vi "Measurement UI.vi"() -> ()   [LabVIEW 2021, in "Waveform Mode_Channel Ganging UI.lvlib"]
uses:
  Waveform Mode_Channel Ganging UI.lvlib
  shared/UI/controls/view.ctl
panel:
  in  "MeasGraphs":enum32{"Results", "Hidden Controls"}(tab)
  in  "Current v/s Time":string="CURRENT v/s TIME"
  in  "Voltage v/s Time":string="VOLTAGE v/s TIME"
  in  "view current legend":T1
  in  "view voltage legend":T1
  out "CurrentGraph":waveform(dbl)[](graph) caption="AC"
  out "VoltageGraph":waveform(dbl)[](graph) caption="AC"
  in  "Mode of operation":T2(ring)
  out "Load dt":dbl[](array[numeric])
  in  "Load source delays":dbl[](array[numeric])
  in  "Load voltage/current setpoints":dbl[](array[numeric]) format="%#_6p"
  in  "Power ON/Source voltage/current setpoints":dbl[](array[numeric]) format="%#_6p"
  in  "Source source delays":dbl[](array[numeric])
  in  "Load voltage/current pole-zero ratios":dbl[](array[numeric])
  in  "Load voltage/current compensation frequencies":dbl[](array[numeric])
  in  "Load voltage/current gain bandwidths":dbl[](array[numeric])
  in  "Source voltage/current pole-zero ratios":dbl[](array[numeric])
  in  "Source voltage/current compensation frequencies":dbl[](array[numeric])
  in  "Source voltage/current gain bandwidths":dbl[](array[numeric])
  in  "Load resource names":string[](array[string])
  in  "Power ON/Source resource names":string[](array[string])
  out "Ganged load currents":dbl[](array[numeric])
  out "Ganged load voltages":dbl[](array[numeric])
  out "Ganged source currents":dbl[](array[numeric])
  out "Ganged source voltages":dbl[](array[numeric])
  out "Load currents":dbl[](array[numeric])
  out "Load voltages":dbl[](array[numeric])
  out "Source currents":dbl[](array[numeric])
  out "Source voltages":dbl[](array[numeric])
  out "Source dt":dbl[](array[numeric])
  in  "ModeOfConfiguration":T3(tab)
  in  "DEVICE POWER":bool=TRUE
  out "Status":string
  in  "Load config power on":string="Load Config"
  in  "POWERON/OFFLOADResourceNames":refnum<k15>[](array[refnum]) caption="RESOURCE NAMES\n(Single/Master & Slave)"
  in  "Source config power on":string="Source Config"
  in  "POWERON/OFFSOURCEResourceNames":refnum<k15>[](array[refnum]) caption="RESOURCE NAMES\n(Single/Master & Slave)"
  in  "Power on/off source sense":i32(ring)=1009 caption="SENSE" items=["Local"=1008, "Remote"=1009]
  in  "Power on/off Source voltage/current limit range":dbl=20.0 caption="CURRENT LIMIT" format="%#_6pA"
  in  "Power on/off Source voltage/current level":dbl=6.0 caption="VOLTAGE LEVEL" format="%#_6pV"
  in  "Power on/off source system configuration":enum32{"Series", "Parallel"}(ring)=enum."Parallel" caption="SYSTEM CONFIG"
  in  "Power on/off output function":i32(ring)=1006 caption="OUTPUT FUNCTION" items=["DC Voltage"=1006, "DC Current"=1007]
  out "Eload status":string
  in  "MeasConfigurations":enum32{"Source Config", "Load Config"}(tab)
  out "Source duration":string="            Duration"
  out "Source voltage/current":string="Voltage"
  in  "Source setpoints":T4(array[cluster]) {"Duration" format="%#_6ps"; "Voltage/Current Value" format="%#_6pV"}
  in  "Source timing":string="Timings"
  in  "Source aperture time":dbl=0.01666 caption="APERTURE TIME" format="%.3ps"
  in  "Source enable/disable":bool=TRUE caption="Source Enable/Disable"
  in  "PPSResourceNames":refnum<k15>[](array[refnum]) caption="RESOURCE NAMES\n(Single/Master & Slave)"
  in  "Source transient response":i32(ring)=1038 caption="TRANSIENT RESPONSE" items=["Slow"=1041, "Normal"=1038, "Fast"=1039, "Custom"=1042]
  in  "Power ON/Source sense":i32(ring)=1009 caption="SENSE" items=["Local"=1008, "Remote"=1009]
  in  "Source voltage/current level range":dbl=20.0 caption="VOLTAGE LEVEL RANGE" format="%#_6pV"
  in  "Source current/voltage limit high":dbl=25.0 caption="CURRENT LIMIT/LIMIT HIGH" format="%#_6pA"
  in  "Power ON/Source current/voltage limit range":dbl=25.0 caption="CURRENT LIMIT RANGE" format="%#_6pA"
  in  "Source limit symmetry":enum32{"Symmetric", "Asymmetric"}(ring)=enum."Asymmetric" caption="LIMIT SYMMETRY"
  in  "Source current/voltage limit low":dbl=-0.6 caption="CURRENT LIMIT LOW" format="%#_6pA"
  in  "Power ON/Source system configuration":enum32{"Series", "Parallel"}(ring)=enum."Parallel" caption="SYSTEM CONFIG"
  in  "Source compliance":string="Compliance"
  in  "Source sourceadapt":string="SourceAdapt"
  in  "Power ON/Source output function":i32(ring)=1006 caption="OUTPUT FUNCTION" items=["DC Voltage"=1006, "DC Current"=1007]
  in  "Source Custom Transient Response":bool
  in  "Load device voltage/current rating":dbl=30.0 caption="MAX CURRENT PER LOAD" format="%#_6pA"
  out "Load duration":string="            Duration"
  out "Load voltage/current":string="Current"
  in  "Load setpoints":T4(array[cluster]) {"Duration" format="%#_6ps"; "Voltage/Current Value" format="%#_6pA"}
  in  "Load aperture time":dbl=0.01666 caption="APERTURE TIME" format="%.3ps"
  in  "Load timing":string="Timings"
  in  "Load Custom Transient Response":bool
  in  "Load sourceadapt":string="SourceAdapt"
  in  "Load compliance":string="Compliance"
  in  "Load system configuration":enum32{"Series", "Parallel"}(ring)=enum."Parallel" caption="SYSTEM CONFIG"
  in  "Load current/voltage limit low":dbl caption="VOLTAGE  LIMIT LOW" format="%#_6pV"
  in  "Load limit symmetry":enum32{"Symmetric", "Asymmetric"}(ring) caption="LIMIT SYMMETRY"
  in  "Load current/voltage limit range":dbl=6.0 caption="VOLTAGE LIMIT RANGE" format="%#_6pV"
  in  "Load current/voltage limit high":dbl=inf caption="VOLTAGE LIMIT/LIMIT HIGH" format="%#_6p"
  in  "Load voltage/current level range":dbl=40.0 caption="CURRENT LEVEL RANGE" format="%#_6pA"
  in  "Load sense":i32(ring)=1009 caption="SENSE" items=["Local"=1008, "Remote"=1009]
  in  "Load transient response":i32(ring)=1038 caption="TRANSIENT RESPONSE" items=["Slow"=1041, "Normal"=1038, "Fast"=1039, "Custom"=1042]
  in  "Load output function":i32(ring)=1007 caption="OUTPUT FUNCTION" items=["DC Voltage"=1006, "DC Current"=1007]
  in  "Load enable/disable":bool caption="Load Enable/Disable"
  in  "LoadResourceNames":refnum<k15>[](array[refnum]) caption="RESOURCE NAMES\n(Single/Master & Slave)"
  # "V"
  # "I"
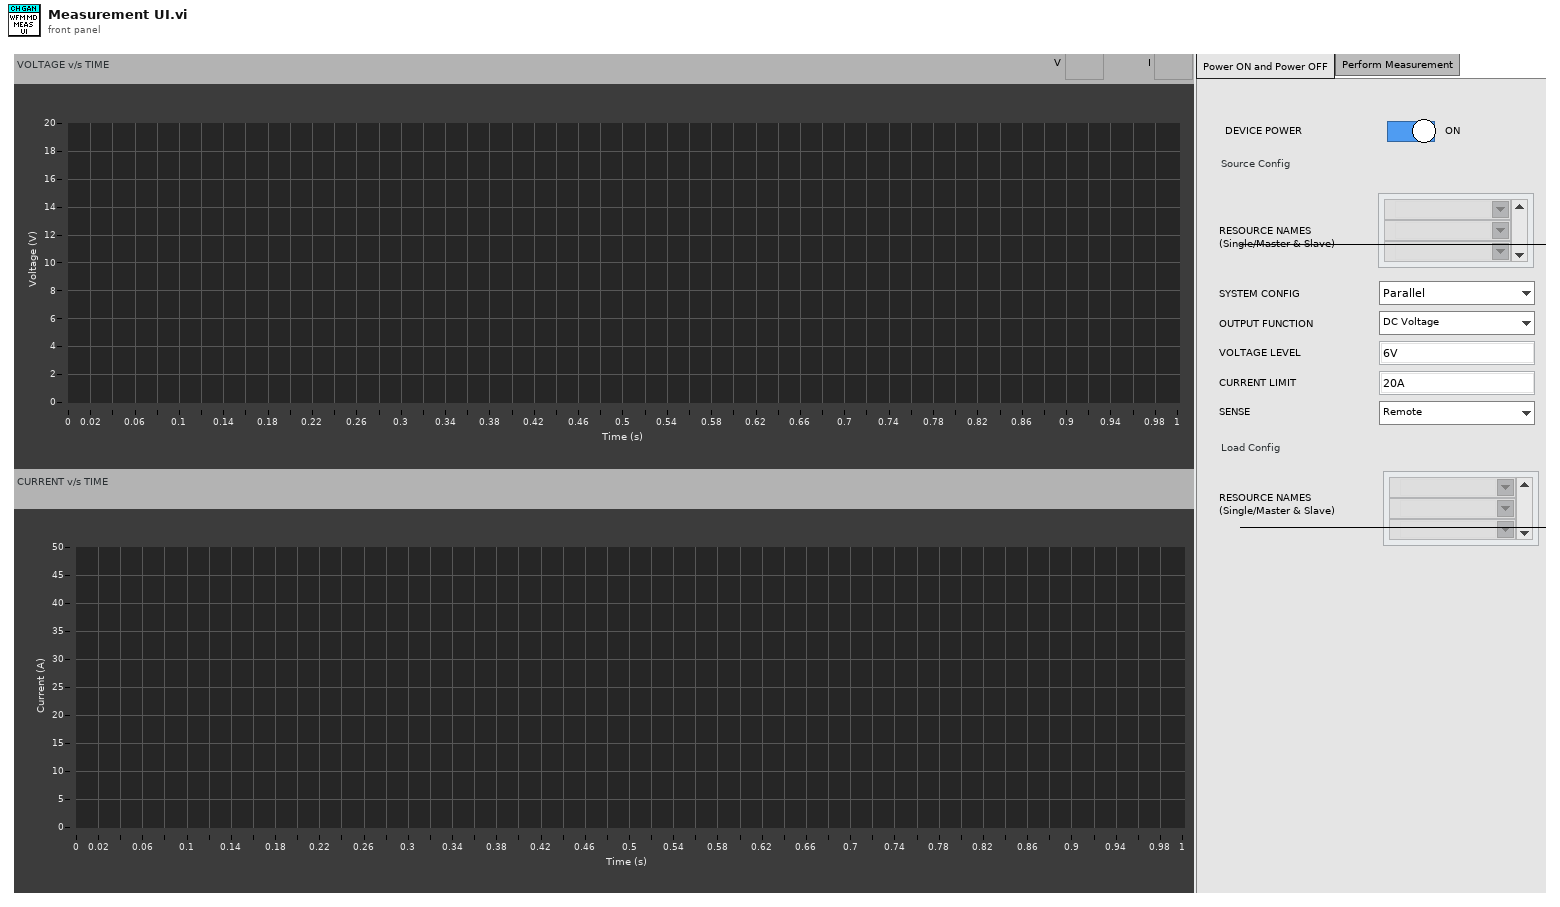
[diagram p1: front panel]
types:
  T1 = typedef "view.ctl" = bool
  T2 = enum32{"Power on the DUT", "Perform measurement", "Power off the DUT"}
  T3 = enum32{"Power ON and Power OFF", "Perform Measurement"}
  T4 = cluster{"Voltage/Current Value":dbl, "Duration":dbl}[]
  T5 = typedef "Multiple SourceAdapt Parameters.ctl" = cluster{"Voltage gain bandwidth":dbl, "Voltage compensation frequency":dbl, "Voltage pole-zero ratio":dbl, "Current gain bandwidth":dbl, "Current compensation frequency":dbl, "Current pole-zero ratio":dbl}[]
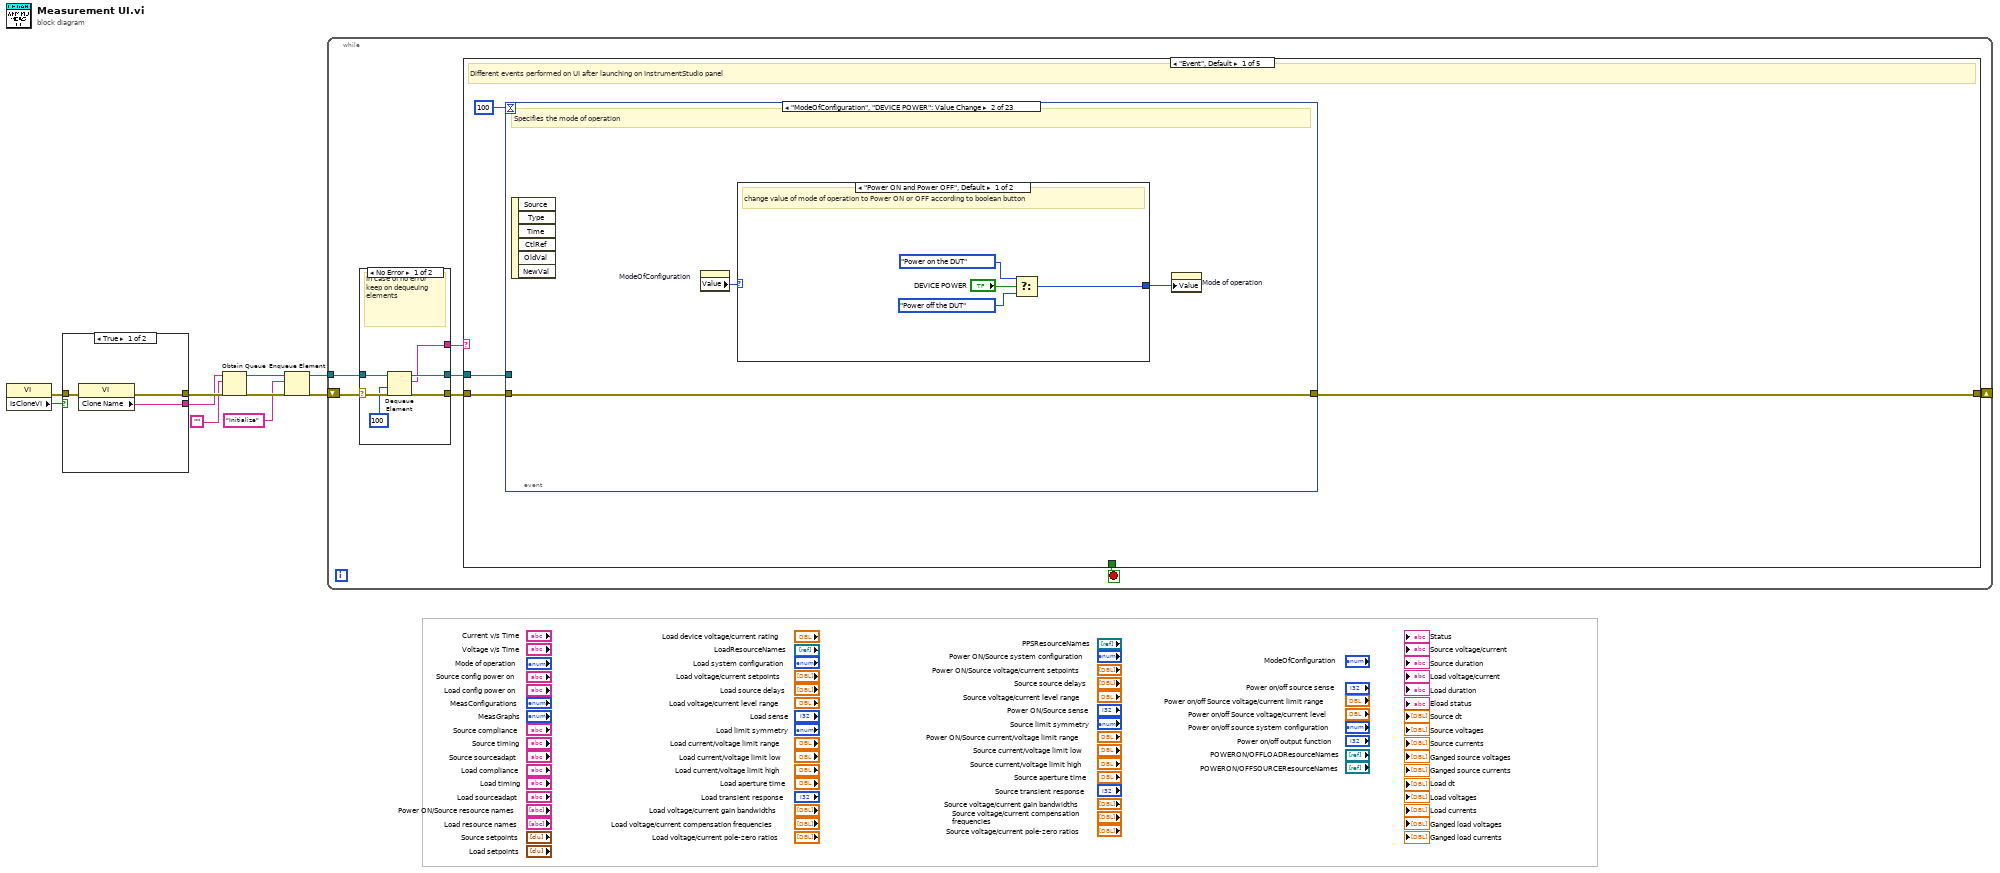
[diagram p0: block diagram]
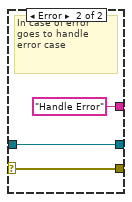
[diagram p2: hidden frame]
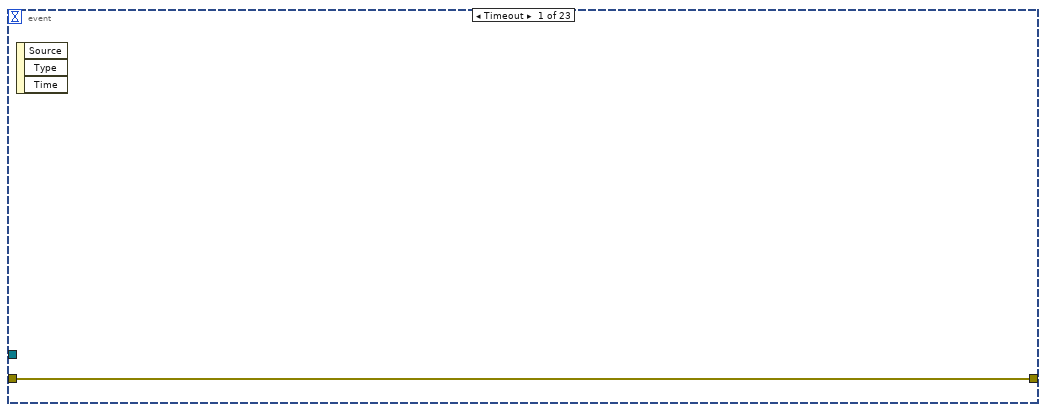
[diagram p3: hidden frame]
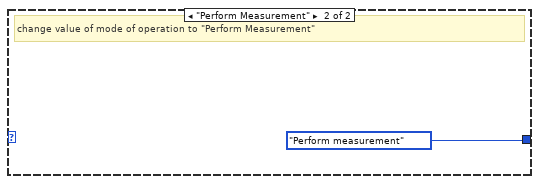
[diagram p4: hidden frame]
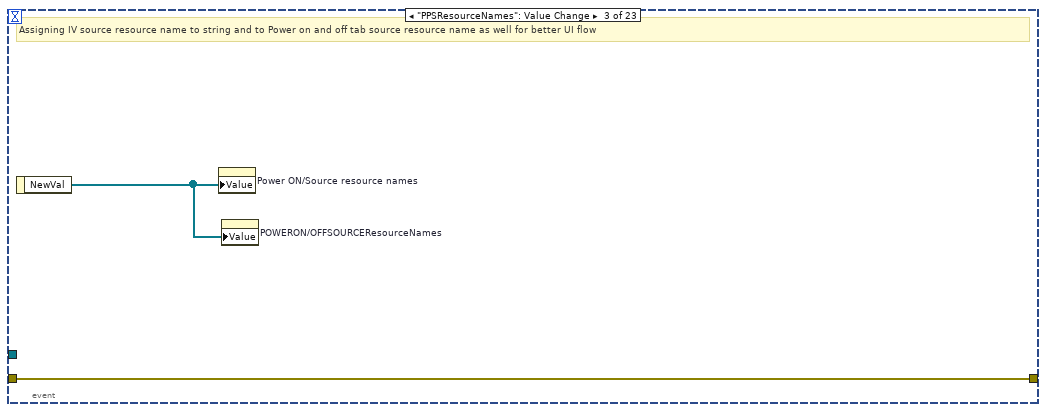
[diagram p5: hidden frame]
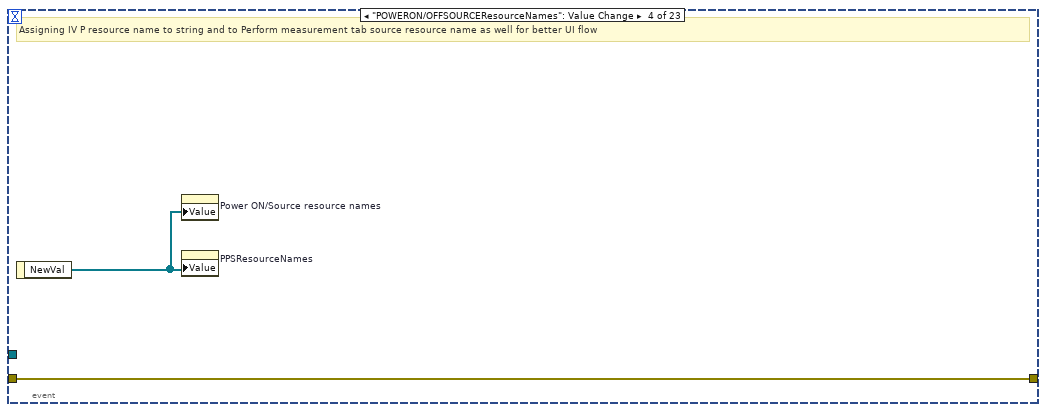
[diagram p6: hidden frame]
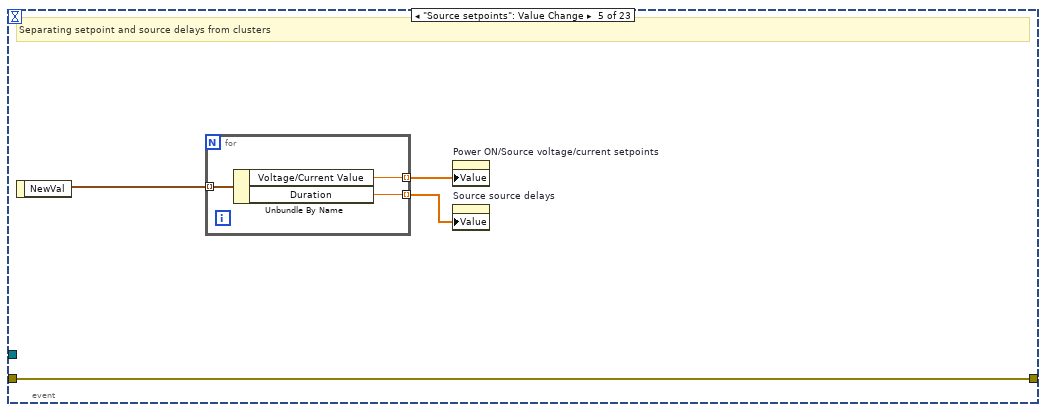
[diagram p7: hidden frame]
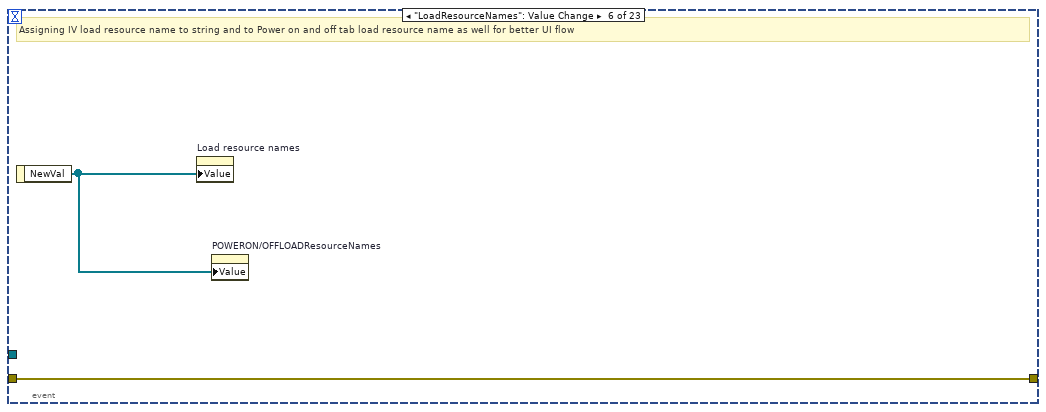
[diagram p8: hidden frame]
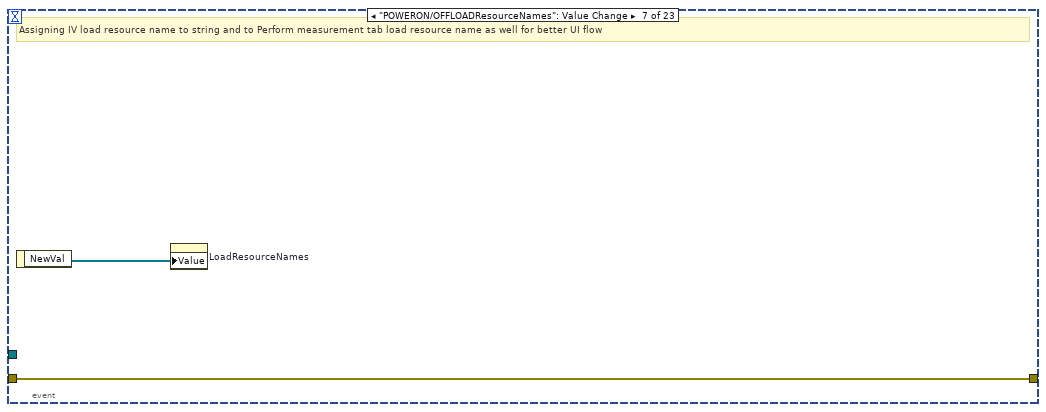
[diagram p9: hidden frame]
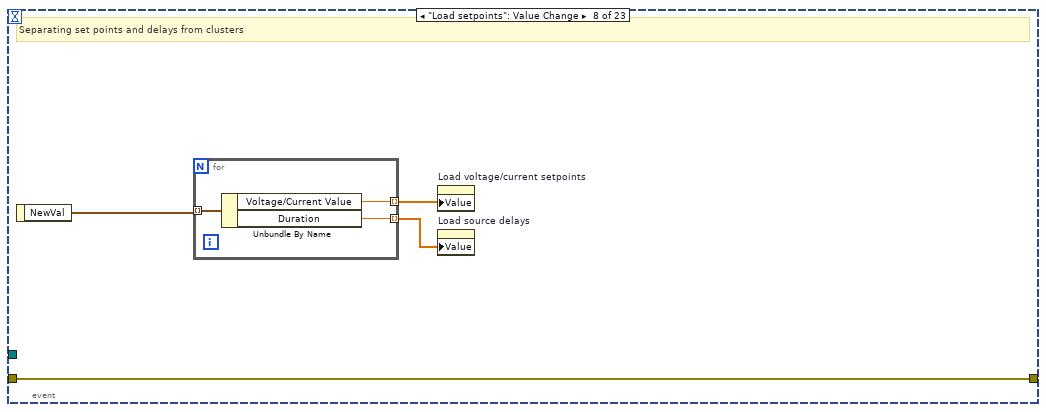
[diagram p10: hidden frame]
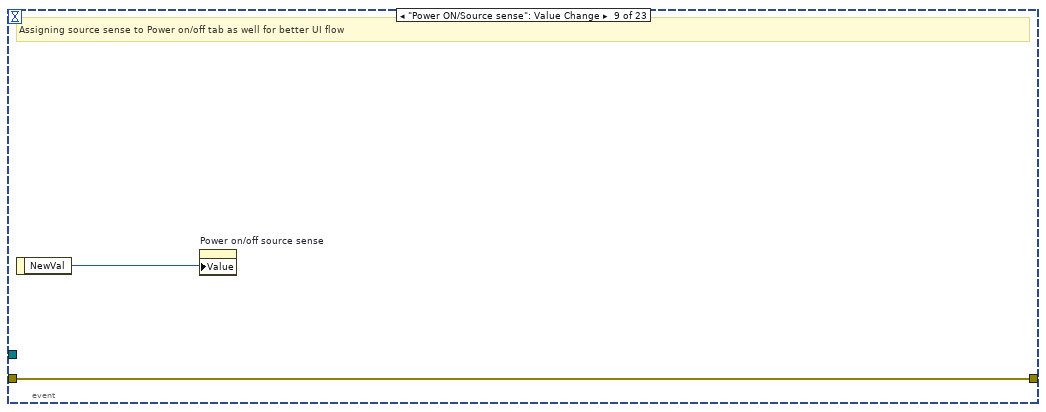
[diagram p11: hidden frame]
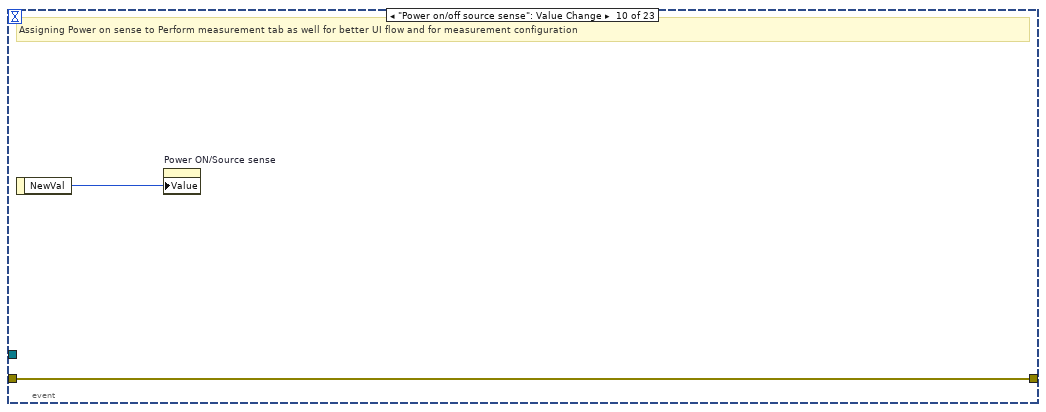
[diagram p12: hidden frame]
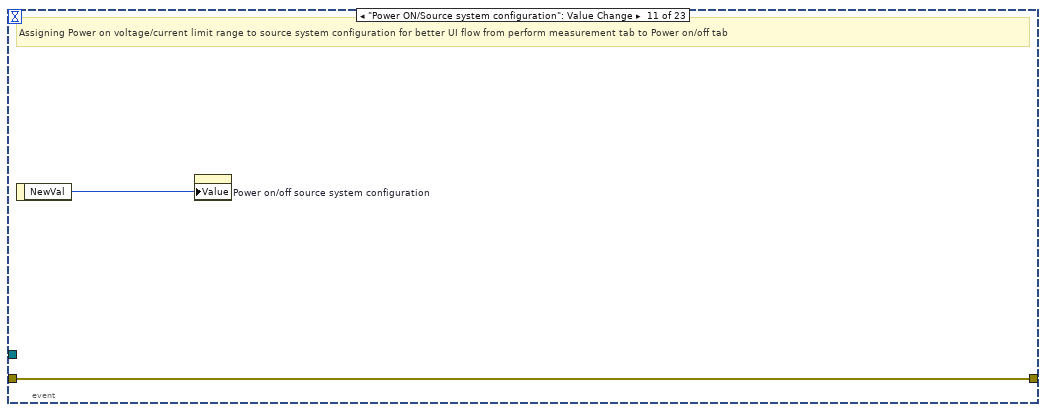
[diagram p13: hidden frame]
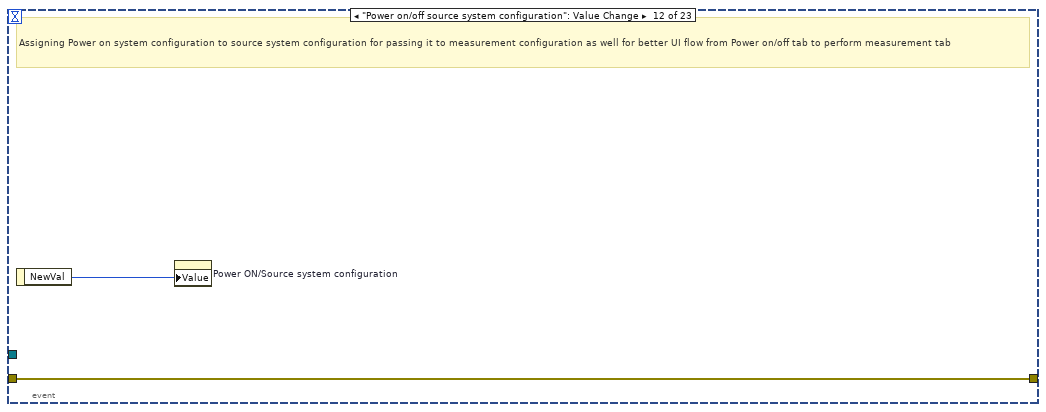
[diagram p14: hidden frame]
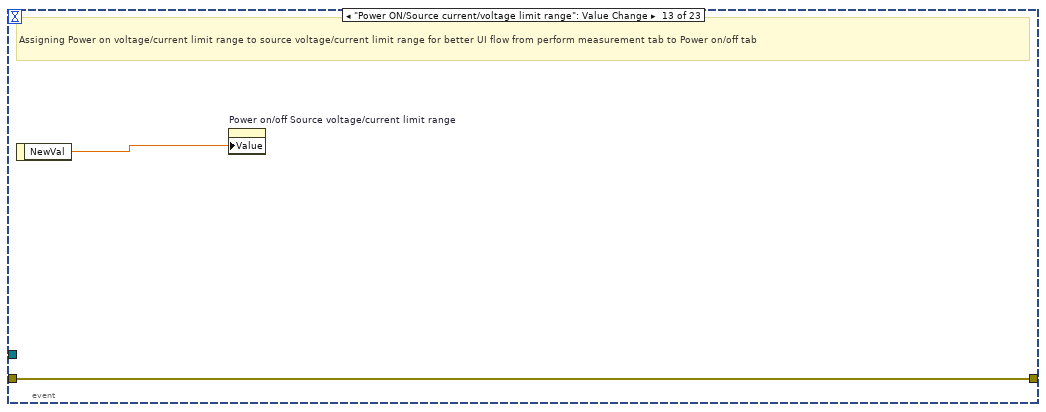
[diagram p15: hidden frame]
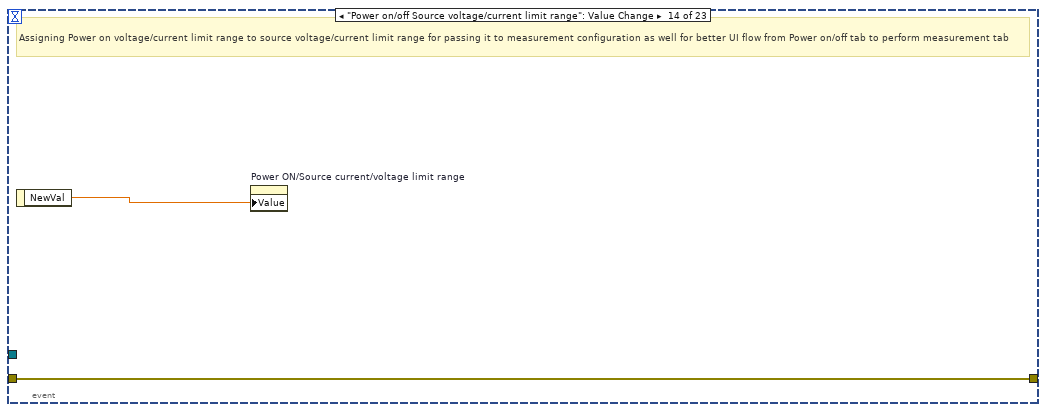
[diagram p16: hidden frame]
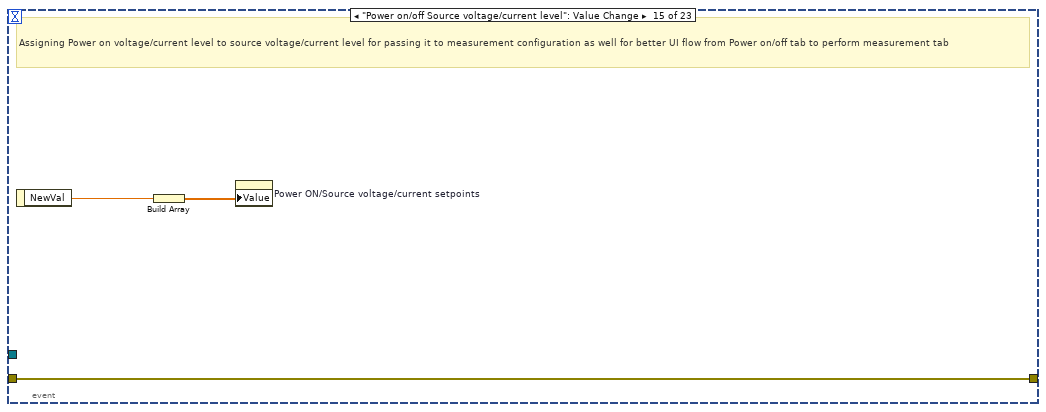
[diagram p17: hidden frame]
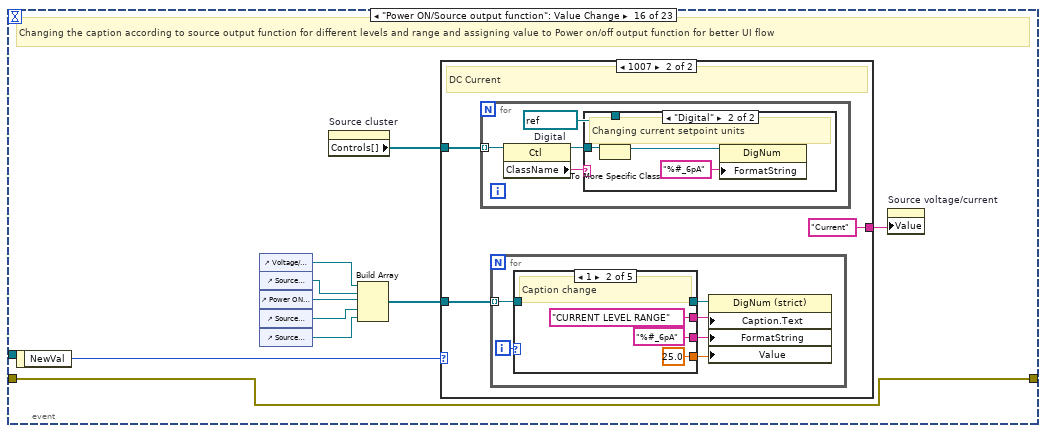
[diagram p18: hidden frame]
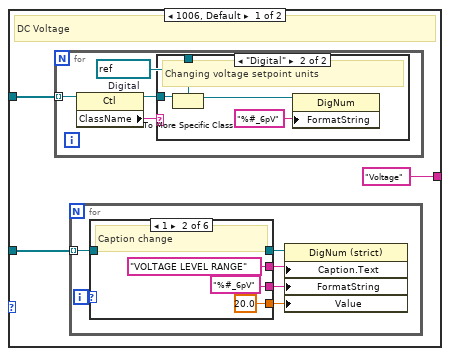
[diagram p19: hidden frame]
diagram:
  n1 = property class="VI"() -> (error out=w1:errorcluster, "IsCloneVI"=w2:bool)  [unwired: 2 in, 1 out]
  n2 = case shown="True" w2 {
    tunnel: [w13 w16] -> w10
    tunnel: [w12 w15] -> w9
    tunnel: w1 -> [w11 w14]
    frame True {
      n3 = property class="VI"(error in=w11) -> (error out=w13:errorcluster, "Clone Name"=w12:string)  [unwired: 1 in, 1 out]
    }
    frame False {
      n4 = property class="VI"(error in=w14) -> (error out=w16:errorcluster, "Name"=w15:string)  [unwired: 1 in, 1 out]
    }
  }
  n5 = Obtain Queue(name (unnamed)=w9, element data type="", error in (no error)=w10) -> (queue out=w6:refnum<queue>, error out=w8:errorcluster)  [unwired: 2 in, 1 out]
  n6 = Enqueue Element(queue=w6, element="Initialize", error in (no error)=w8) -> (queue out=w5:refnum<queue>, error out=w7:errorcluster)  [unwired: 1 in, 1 out]
  n7 = while {
    shift-right: [w18] -> _
    shift-left: w7 -> [w23]
    tunnel: w5 -> [w21]
    stop <- w17 stop-if-true
    n8 = case shown="No Error" w23 {
      selector: w23 -> [w29 w32]
      tunnel: [w28 w32] -> w22
      tunnel: w21 -> [w27 w31]
      tunnel: [w26 w31] -> w20
      tunnel: [w25 "Handle Error"] -> w19
      frame No Error {
        # "In case of no error keep on dequeuing elements"
        n9 = Dequeue Element(queue=w27, timeout in ms (-1)=100, error in (no error)=w29) -> (queue out=w26:refnum<queue>, element=w25:string, error out=w28:errorcluster)  [unwired: 1 out]
      }
      frame Error {
        # "In case of error goes to handle error case"
      }
    }
    n10 = case shown="\"Event\", Default" w19 {
      tunnel: w22 -> [w35 w348 w376 w470 w471]
      tunnel: w20 -> [w33 _ _ w468 _]
      tunnel: [w36 w348 w376 w465 w471] -> w18
      tunnel: [_ _ _ TRUE _] -> w17
      frame "Event", Default {
        # "Different events performed on UI after launching on InstrumentStudio panel"
        n11 = event shown="[1] \"ModeOfConfiguration\", \"DEVICE POWER\": Value Change" {
          selector: _ -> [_ _ _ _ _ _ _ _ _ _ _ _ _ _ _ _ _ _ _ _ _ _ _]
          dyn-events: _ -> [_ _ _ _ _ _ _ _ _ _ _ _ _ _ _ _ _ _ _ _ _ _ _]
          timeout: 100 -> [_ _ _ _ _ _ _ _ _ _ _ _ _ _ _ _ _ _ _ _ _ _ _]
          tunnel: [w37 w38 w47 w48 w52 w58 w59 w63 w68 w70 w72 w74 w76 w78 w80 w83 w165 w200 w286 w305 w319 w332 w345] -> w36
          tunnel: w35 -> [w37 w38 w47 w48 w52 w58 w59 w63 w68 w70 w72 w74 w76 w78 w80 w83 w165 w200 w286 w305 w320 w333 w346]
          tunnel: w33 -> [_ _ _ _ _ _ _ _ _ _ _ _ _ _ _ _ _ _ _ _ _ _ w344]
          event Timeout {
            n12 = event-data() -> ()  [unwired: 1 in, 3 out]
          }
          event "ModeOfConfiguration", "DEVICE POWER": Value Change {
            # "Specifies the mode of operation"
            n13 = event-data() -> ()  [unwired: 1 in, 6 out]
            n14 = property on="ModeOfConfiguration" class="TabCtl (strict)"() -> ("Value"=w40:T3)  [unwired: 2 in, 2 out]
            n15 = case shown="\"Power ON and Power OFF\", Default" w40 {
              tunnel: [w42 T2."Perform measurement" ("Mode of operation")] -> w39
              frame "Power ON and Power OFF", Default {
                # "change value of mode of operation to Power ON or OFF according to boolean button"
                n16 = Select(t=T2."Power on the DUT" ("Mode of operation"), s="DEVICE POWER", f=T2."Power off the DUT" ("Mode of operation")) -> (s? t:f=w42:T2)
              }
              frame "Perform Measurement" {
                # "change value of mode of operation to \"Perform Measurement\""
              }
            }
            n17 = property on="Mode of operation" class="Enum (strict)"("Value"=w39) -> ()  [unwired: 2 in, 2 out]
          }
          event "PPSResourceNames": Value Change {
            # "Assigning IV source resource name to string and to Power on and off tab source resource name as well for better UI flow"
            n18 = event-data() -> ("NewVal"=w46:refnum<k15>[])  [unwired: 1 in]
            n19 = property on="Power ON/Source resource names" class="Arr (strict)"("Value"=w46) -> ()  [unwired: 2 in, 2 out]
            n20 = property on="POWERON/OFFSOURCEResourceNames" class="Arr (strict)"("Value"=w46) -> ()  [unwired: 2 in, 2 out]
          }
          event "POWERON/OFFSOURCEResourceNames": Value Change {
            # "Assigning IV P resource name to string and to Perform measurement tab source resource name as well for better UI flow"
            n21 = event-data() -> ("NewVal"=w49:refnum<k15>[])  [unwired: 1 in]
            n22 = property on="Power ON/Source resource names" class="Arr (strict)"("Value"=w49) -> ()  [unwired: 2 in, 2 out]
            n23 = property on="PPSResourceNames" class="Arr (strict)"("Value"=w49) -> ()  [unwired: 2 in, 2 out]
          }
          event "Source setpoints": Value Change {
            # "Separating setpoint and source delays from clusters"
            n24 = event-data() -> ("NewVal"=w53:T4)  [unwired: 1 in]
            n25 = for {
              tunnel: w53 -> [w56] mode=indexing
              tunnel: [w55] -> w51 mode=indexing
              tunnel: [w54] -> w50 mode=indexing
              n26 = Unbundle By Name(w56) -> ("Voltage/Current Value"=w55:dbl, "Duration"=w54:dbl)
            }
            n27 = property on="Power ON/Source voltage/current setpoints" class="Arr (strict)"("Value"=w51) -> ()  [unwired: 2 in, 2 out]
            n28 = property on="Source source delays" class="Arr (strict)"("Value"=w50) -> ()  [unwired: 2 in, 2 out]
          }
          event "LoadResourceNames": Value Change {
            # "Assigning IV load resource name to string and to Power on and off tab load resource name as well for better UI flow"
            n29 = event-data() -> ("NewVal"=w57:refnum<k15>[])  [unwired: 1 in]
            n30 = property on="Load resource names" class="Arr (strict)"("Value"=w57) -> ()  [unwired: 2 in, 2 out]
            n31 = property on="POWERON/OFFLOADResourceNames" class="Arr (strict)"("Value"=w57) -> ()  [unwired: 2 in, 2 out]
          }
          event "POWERON/OFFLOADResourceNames": Value Change {
            # "Assigning IV load resource name to string and to Perform measurement tab load resource name as well for better UI flow"
            n32 = event-data() -> ("NewVal"=w60:refnum<k15>[])  [unwired: 1 in]
            n33 = property on="LoadResourceNames" class="Arr (strict)"("Value"=w60) -> ()  [unwired: 2 in, 2 out]
          }
          event "Load setpoints": Value Change {
            # "Separating set points and delays from clusters"
            n34 = event-data() -> ("NewVal"=w64:T4)  [unwired: 1 in]
            n35 = for {
              tunnel: w64 -> [w67] mode=indexing
              tunnel: [w66] -> w62 mode=indexing
              tunnel: [w65] -> w61 mode=indexing
              n36 = Unbundle By Name(w67) -> ("Voltage/Current Value"=w66:dbl, "Duration"=w65:dbl)
            }
            n37 = property on="Load voltage/current setpoints" class="Arr (strict)"("Value"=w62) -> ()  [unwired: 2 in, 2 out]
            n38 = property on="Load source delays" class="Arr (strict)"("Value"=w61) -> ()  [unwired: 2 in, 2 out]
          }
          event "Power ON/Source sense": Value Change {
            # "Assigning source sense to Power on/off tab as well for better UI flow"
            n39 = event-data() -> ("NewVal"=w69:i32)  [unwired: 1 in]
            n40 = property on="Power on/off source sense" class="Ring (strict)"("Value"=w69) -> ()  [unwired: 2 in, 2 out]
          }
          event "Power on/off source sense": Value Change {
            # "Assigning Power on sense to Perform measurement tab as well for better UI flow and for measurement configuration"
            n41 = event-data() -> ("NewVal"=w71:i32)  [unwired: 1 in]
            n42 = property on="Power ON/Source sense" class="Ring (strict)"("Value"=w71) -> ()  [unwired: 2 in, 2 out]
          }
          event "Power ON/Source system configuration": Value Change {
            # "Assigning Power on voltage/current limit range to source system configuration for better UI flow from perform measurement tab to Power on/off tab"
            n43 = event-data() -> ("NewVal"=w73:enum32{"Series", "Parallel"})  [unwired: 1 in]
            n44 = property on="Power on/off source system configuration" class="Enum (strict)"("Value"=w73) -> ()  [unwired: 2 in, 2 out]
          }
          event "Power on/off source system configuration": Value Change {
            # "Assigning Power on system configuration to source system configuration for passing it to measurement configuration as well for better UI flow from Power on/off tab to perform measurement tab"
            n45 = event-data() -> ("NewVal"=w75:enum32{"Series", "Parallel"})  [unwired: 1 in]
            n46 = property on="Power ON/Source system configuration" class="Enum (strict)"("Value"=w75) -> ()  [unwired: 2 in, 2 out]
          }
          event "Power ON/Source current/voltage limit range": Value Change {
            # "Assigning Power on voltage/current limit range to source voltage/current limit range for better UI flow from perform measurement tab to Power on/off tab"
            n47 = event-data() -> ("NewVal"=w77:dbl)  [unwired: 1 in]
            n48 = property on="Power on/off Source voltage/current limit range" class="DigNum (strict)"("Value"=w77) -> ()  [unwired: 2 in, 2 out]
          }
          event "Power on/off Source voltage/current limit range": Value Change {
            # "Assigning Power on voltage/current limit range to source voltage/current limit range for passing it to measurement configuration as well for better UI flow from Power on/off tab to perform measurement tab"
            n49 = event-data() -> ("NewVal"=w79:dbl)  [unwired: 1 in]
            n50 = property on="Power ON/Source current/voltage limit range" class="DigNum (strict)"("Value"=w79) -> ()  [unwired: 2 in, 2 out]
          }
          event "Power on/off Source voltage/current level": Value Change {
            # "Assigning Power on voltage/current level to source voltage/current level for passing it to measurement configuration as well for better UI flow from Power on/off tab to perform measurement tab"
            n51 = event-data() -> ("NewVal"=w82:dbl)  [unwired: 1 in]
            n52 = Build Array(w82) -> (w81:dbl[])
            n53 = property on="Power ON/Source voltage/current setpoints" class="Arr (strict)"("Value"=w81) -> ()  [unwired: 2 in, 2 out]
          }
          event "Power ON/Source output function": Value Change {
            # "Changing the caption according to source output function for different levels and range and assigning value to Power on/off output function for better UI flow"
            n54 = event-data() -> ("NewVal"=w92:i32)  [unwired: 1 in]
            n55 = control-ref of="Voltage/Current Value"() -> (w86:refnum<vi>)
            n56 = control-ref of="Source voltage/current level range"() -> (w91:refnum<vi>)
            n57 = control-ref of="Power ON/Source current/voltage limit range"() -> (w90:refnum<vi>)
            n58 = control-ref of="Source current/voltage limit low"() -> (w89:refnum<vi>)
            n59 = control-ref of="Source current/voltage limit high"() -> (w88:refnum<vi>)
            n60 = property on="Source cluster" class="Clust (strict)"() -> ("Controls[]"=w85:refnum<vi>[])  [unwired: 2 in, 2 out]
            n61 = Build Array(w86, w91, w90, w89, w88) -> (w87:refnum<vi>[])
            n62 = case shown="1007" w92 {
              tunnel: w87 -> [w95 w129]
              tunnel: w85 -> [w94 w128]
              tunnel: ["Voltage" ("Source voltage/current") "Current" ("Source voltage/current")] -> w84
              frame 1006, Default {
                # "DC Voltage"
                n63 = for {
                  tunnel: w94 -> [w99] mode=indexing
                  w97 = refnum<vi> refnum  # Digital
                  n64 = property class="Ctl"(reference=w99) -> (reference out=w98:refnum<vi>, "ClassName"=w96:string)  [unwired: 1 in, 1 out]
                  n65 = case shown="\"Digital\"" w96 {
                    tunnel: w98 -> [_ w103]
                    tunnel: w97 -> [_ w102]
                    frame Default {
                    }
                    frame "Digital" {
                      # "Changing voltage setpoint units"
                      n66 = To More Specific Class(target class=w102, reference=w103) -> (specific class reference=w101:refnum<vi>)  [unwired: 1 in, 1 out]
                      n67 = property class="DigNum"(reference=w101, "FormatString"="%#_6pV" ("Format String")) -> ()  [unwired: 1 in, 2 out]
                    }
                  }
                }
                n68 = for {
                  tunnel: w95 -> [w107] mode=indexing
                  i -> [w109]
                  n69 = case shown="1" w109 {
                    tunnel: [w110 w114 w118 w121 w125 _] -> w108
                    tunnel: w107 -> [w110 w114 w118 w121 w125 _]
                    tunnel: [_ "VOLTAGE LEVEL RANGE" ("Caption.Text") "CURRENT LIMIT RANGE" ("Caption.Text") "CURRENT LIMIT LOW" ("Caption.Text") "CURRENT LIMIT/LIMIT HIGH" ("Caption.Text") _] -> w106
                    tunnel: [_ "%#_6pV" ("Format String") "%#_6pA" ("Format String") "%#_6pA" ("Format String") "%#_6pA" ("Format String") _] -> w105
                    tunnel: [_ 20.0 ("Value") 25.0 ("Value") -0.6 ("Value") 25.0 ("Value") _] -> w104
                    frame 0 {
                    }
                    frame 1 {
                      # "Caption change"
                    }
                    frame 2 {
                      # "Caption change"
                    }
                    frame 3 {
                      # "Caption change"
                    }
                    frame 4 {
                      # "Caption change"
                    }
                    frame Default {
                    }
                  }
                  n70 = property class="DigNum (strict)"(reference=w108, "Caption.Text"=w106, "FormatString"=w105, "Value"=w104) -> ()  [unwired: 1 in, 2 out]
                }
              }
              frame 1007 {
                # "DC Current"
                n71 = for {
                  tunnel: w128 -> [w133] mode=indexing
                  w131 = refnum<vi> refnum  # Digital
                  n72 = property class="Ctl"(reference=w133) -> (reference out=w132:refnum<vi>, "ClassName"=w130:string)  [unwired: 1 in, 1 out]
                  n73 = case shown="\"Digital\"" w130 {
                    tunnel: w132 -> [_ w137]
                    tunnel: w131 -> [_ w136]
                    frame Default {
                    }
                    frame "Digital" {
                      # "Changing current setpoint units"
                      n74 = To More Specific Class(target class=w136, reference=w137) -> (specific class reference=w135:refnum<vi>)  [unwired: 1 in, 1 out]
                      n75 = property class="DigNum"(reference=w135, "FormatString"="%#_6pA" ("Format String")) -> ()  [unwired: 1 in, 2 out]
                    }
                  }
                }
                n76 = for {
                  tunnel: w129 -> [w141] mode=indexing
                  i -> [w143]
                  n77 = case shown="1" w143 {
                    tunnel: [w144 w148 w152 w155 w159] -> w142
                    tunnel: w141 -> [w144 w148 w152 w155 w159]
                    tunnel: [_ "CURRENT LEVEL RANGE" ("Caption.Text") "VOLTAGE LIMIT RANGE" ("Caption.Text") "VOLTAGE  LIMIT LOW" ("Caption.Text") "VOLTAGE LIMIT/LIMIT HIGH" ("Caption.Text")] -> w140
                    tunnel: [_ "%#_6pA" ("Format String") "%#_6pV" ("Format String") "%#_6pV" ("Format String") "%#_6pV" ("Format String")] -> w139
                    tunnel: [_ 25.0 ("Value") 20.0 ("Value") -0.6 ("Value") 20.0 ("Value")] -> w138
                    frame 0, Default {
                    }
                    frame 1 {
                      # "Caption change"
                    }
                    frame 2 {
                      # "Caption change"
                    }
                    frame 3 {
                      # "Caption change"
                    }
                    frame 4 {
                      # "Caption change"
                    }
                  }
                  n78 = property class="DigNum (strict)"(reference=w142, "Caption.Text"=w140, "FormatString"=w139, "Value"=w138) -> ()  [unwired: 1 in, 2 out]
                }
              }
            }
            n79 = property on="Source voltage/current" class="Str"("Value"=w84) -> ()  [unwired: 2 in, 2 out]
          }
          event "Power on/off output function": Value Change {
            # "Assigning Power on output function to source output function for passing it to measurement configuration as well for better UI flow"
            n80 = event-data() -> ("NewVal"=w164:i32)  [unwired: 1 in]
            n81 = property on="Power ON/Source output function" class="Ring (strict)"("Value"=w164) -> ()  [unwired: 2 in, 2 out]
            n82 = control-ref of="Power on/off Source voltage/current level"() -> (w161:refnum<vi>)
            n83 = control-ref of="Power on/off Source voltage/current limit range"() -> (w162:refnum<vi>)
            n84 = Build Array(w162, w161) -> (w163:refnum<vi>[])
            n85 = case shown="1006, Default" w164 {
              tunnel: w163 -> [w167 w184]
              tunnel: [w166 w183] -> _
              frame 1006, Default {
                # "DC Voltage"
                n86 = for {
                  tunnel: w167 -> [w172] mode=indexing
                  tunnel: [w168] -> w166 mode=indexing
                  i -> [w174]
                  n87 = case shown="0, 2" w174 {
                    tunnel: [w178 w182 _] -> w173
                    tunnel: w172 -> [w178 w182 _]
                    tunnel: ["VOLTAGE LEVEL" ("Caption.Text") "CURRENT LIMIT" ("Caption.Text") _] -> w171
                    tunnel: ["%#_6pV" ("Format String") "%#_6pA" ("Format String") _] -> w170
                    tunnel: [6.0 ("Value") 20.0 ("Value") _] -> w169
                    frame 1 {
                      # "Voltage level cap change"
                    }
                    frame 0, 2 {
                      # "Current limit cap change"
                    }
                    frame Default {
                    }
                  }
                  n88 = property class="DigNum (strict)"(reference=w173, "Caption.Text"=w171, "FormatString"=w170, "Value"=w169) -> (reference out=w168:refnum<vi>)  [unwired: 1 in, 1 out]
                }
              }
              frame 1007 {
                # "DC Current"
                n89 = for {
                  tunnel: w184 -> [w189] mode=indexing
                  tunnel: [w185] -> w183 mode=indexing
                  i -> [w191]
                  n90 = case shown="1" w191 {
                    tunnel: [w195 w199 _] -> w190
                    tunnel: w189 -> [w195 w199 _]
                    tunnel: ["CURRENT LEVEL" ("Caption.Text") "VOLTAGE LIMIT" ("Caption.Text") _] -> w188
                    tunnel: ["%#_6pA" ("Format String") "%#_6pV" ("Format String") _] -> w187
                    tunnel: [10.0 ("Value") 20.0 ("Value") _] -> w186
                    frame 1 {
                      # "Current level cap change"
                    }
                    frame 0, 2 {
                      # "Voltage limit cap change"
                    }
                    frame Default {
                    }
                  }
                  n91 = property class="DigNum (strict)"(reference=w190, "Caption.Text"=w188, "FormatString"=w187, "Value"=w186) -> (reference out=w185:refnum<vi>)  [unwired: 1 in, 1 out]
                }
              }
            }
          }
          event "Load output function": Value Change {
            # "Changing reference according to Load output function DC Current or DC voltage"
            n92 = event-data() -> ("NewVal"=w201:i32)  [unwired: 1 in]
            n93 = property on="Power on/off output function" class="Ring (strict)"("Value"=w201) -> ()  [unwired: 2 in, 2 out]
            n94 = control-ref of="Voltage/Current Value"() -> (w204:refnum<vi>)
            n95 = control-ref of="Load voltage/current level range"() -> (w209:refnum<vi>)
            n96 = control-ref of="Load current/voltage limit range"() -> (w208:refnum<vi>)
            n97 = control-ref of="Load current/voltage limit low"() -> (w207:refnum<vi>)
            n98 = control-ref of="Load current/voltage limit high"() -> (w206:refnum<vi>)
            n99 = property on="Load cluster" class="Clust (strict)"() -> ("Controls[]"=w203:refnum<vi>[])  [unwired: 2 in, 2 out]
            n100 = Build Array(w204, w209, w208, w207, w206) -> (w205:refnum<vi>[])
            n101 = case shown="1007, Default" w201 {
              tunnel: w205 -> [w213 w248]
              tunnel: w203 -> [w211 w246]
              tunnel: ["Voltage" ("Load voltage/current") "Current" ("Load voltage/current")] -> w202
              frame 1006 {
                # "DC Voltage"
                n102 = for {
                  N: 1 -> [_]
                  tunnel: w211 -> [w217] mode=indexing
                  w215 = refnum<vi> refnum  # Digital
                  n103 = property class="Ctl"(reference=w217) -> (reference out=w216:refnum<vi>, "ClassName"=w214:string)  [unwired: 1 in, 1 out]
                  n104 = case shown="\"Digital\"" w214 {
                    tunnel: w216 -> [_ w221]
                    tunnel: w215 -> [_ w220]
                    frame Default {
                    }
                    frame "Digital" {
                      # "Changing voltage setpoint units"
                      n105 = To More Specific Class(target class=w220, reference=w221) -> (specific class reference=w219:refnum<vi>)  [unwired: 1 in, 1 out]
                      n106 = property class="DigNum"(reference=w219, "FormatString"="%#_6pV" ("Format String")) -> ()  [unwired: 1 in, 2 out]
                    }
                  }
                }
                n107 = for {
                  tunnel: w213 -> [w225] mode=indexing
                  i -> [w227]
                  n108 = case shown="1" w227 {
                    tunnel: [w228 w232 w236 w239 w243 _] -> w226
                    tunnel: w225 -> [w228 w232 w236 w239 w243 _]
                    tunnel: [_ "VOLTAGE LEVEL RANGE" ("Caption.Text") "CURRENT LIMIT RANGE" ("Caption.Text") "CURRENT LIMIT LOW" ("Caption.Text") "CURRENT LIMIT/LIMIT HIGH" ("Caption.Text") _] -> w224
                    tunnel: [_ "%#_6pV" ("Format String") "%#_6pA" ("Format String") "%#_6pA" ("Format String") "%#_6pA" ("Format String") _] -> w223
                    tunnel: [_ 6.0 ("Value") 40.0 ("Value") 0.0 ("Value") 40.0 ("Value") _] -> w222
                    frame 0 {
                    }
                    frame 1 {
                      # "Caption change"
                    }
                    frame 2 {
                      # "Caption change"
                    }
                    frame 3 {
                      # "Caption change"
                    }
                    frame 4 {
                      # "Caption change"
                    }
                    frame Default {
                    }
                  }
                  n109 = property class="DigNum (strict)"(reference=w226, "Caption.Text"=w224, "FormatString"=w223, "Value"=w222) -> ()  [unwired: 1 in, 2 out]
                }
              }
              frame 1007, Default {
                # "DC Current"
                n110 = for {
                  N: 1 -> [_]
                  tunnel: w246 -> [w252] mode=indexing
                  w250 = refnum<vi> refnum  # Digital
                  n111 = property class="Ctl"(reference=w252) -> (reference out=w251:refnum<vi>, "ClassName"=w249:string)  [unwired: 1 in, 1 out]
                  n112 = case shown="\"Digital\"" w249 {
                    tunnel: w251 -> [_ w256]
                    tunnel: w250 -> [_ w255]
                    frame Default {
                    }
                    frame "Digital" {
                      # "Changing current setpoint units"
                      n113 = To More Specific Class(target class=w255, reference=w256) -> (specific class reference=w254:refnum<vi>)  [unwired: 1 in, 1 out]
                      n114 = property class="DigNum"(reference=w254, "FormatString"="%#_6pA" ("Format String")) -> ()  [unwired: 1 in, 2 out]
                    }
                  }
                }
                n115 = for {
                  tunnel: w248 -> [w260] mode=indexing
                  i -> [w262]
                  n116 = case shown="1" w262 {
                    tunnel: [w263 w267 w271 w274 w279 _] -> w261
                    tunnel: w260 -> [w263 w267 w271 w274 w279 _]
                    tunnel: [_ "CURRENT LEVEL RANGE" ("Caption.Text") "VOLTAGE LIMIT RANGE" ("Caption.Text") "VOLTAGE  LIMIT LOW" ("Caption.Text") "VOLTAGE LIMIT/LIMIT HIGH" ("Caption.Text") _] -> w259
                    tunnel: [_ "%#_6pA" ("Format String") "%#_6pV" ("Format String") "%#_6pV" ("Format String") "%#_6p" ("Format String") _] -> w258
                    tunnel: [_ 40.0 ("Value") 6.0 ("Value") 0.0 ("Value") w277 _] -> w257
                    frame 0 {
                    }
                    frame 1 {
                      # "Caption change"
                    }
                    frame 2 {
                      # "Caption change"
                    }
                    frame 3 {
                      # "Caption change"
                    }
                    frame 4 {
                      # "Caption change"
                      n117 = Reciprocal(x=0.0) -> (1/x=w277:dbl)
                    }
                    frame Default {
                    }
                  }
                  n118 = property class="DigNum (strict)"(reference=w261, "Caption.Text"=w259, "FormatString"=w258, "Value"=w257) -> ()  [unwired: 1 in, 2 out]
                }
              }
            }
            n119 = property on="Load voltage/current" class="Str"("Value"=w202) -> ()  [unwired: 2 in, 2 out]
          }
          event "Source Custom Transient Response": Value Change {
            # "Custom transienet response protiestins assignment"
            n120 = event-data() -> ()  [unwired: 1 in, 5 out]
            n121 = call "Custom Transient Response for Setpoints.vi"() -> ("SourceAdapt Parameters"=w285:T5)  [unwired: 11 in]
            n122 = for {
              tunnel: w285 -> [w291] mode=indexing
              tunnel: "Power ON/Source output function" -> [w290]
              tunnel: [w289] -> w283 mode=indexing
              tunnel: [w288] -> w282 mode=indexing
              tunnel: [w287] -> w281 mode=indexing
              n123 = case shown="1007" w290 {
                tunnel: w291 -> [w295 w299]
                tunnel: [w294 w297] -> w289
                tunnel: [w293 w298] -> w288
                tunnel: [w292 w296] -> w287
                frame 1007 {
                  # "DC Current"
                  n124 = Unbundle By Name(w295) -> ("Current gain bandwidth"=w293:dbl, "Current compensation frequency"=w294:dbl, "Current pole-zero ratio"=w292:dbl)
                }
                frame 1006, Default {
                  # "DC Voltage"
                  n125 = Unbundle By Name(w299) -> ("Voltage gain bandwidth"=w298:dbl, "Voltage compensation frequency"=w297:dbl, "Voltage pole-zero ratio"=w296:dbl)
                }
              }
            }
            n126 = property on="Source voltage/current gain bandwidths" class="Arr (strict)"("Value"=w282) -> ()  [unwired: 2 in, 2 out]
            n127 = property on="Source voltage/current compensation frequencies" class="Arr (strict)"("Value"=w283) -> ()  [unwired: 2 in, 2 out]
            n128 = property on="Source voltage/current pole-zero ratios" class="Arr (strict)"("Value"=w281) -> ()  [unwired: 2 in, 2 out]
          }
          event "Load Custom Transient Response": Value Change {
            # "Custom transienet response protiestins assignment"
            n129 = event-data() -> ()  [unwired: 1 in, 5 out]
            n130 = call "Custom Transient Response for Setpoints.vi"() -> ("SourceAdapt Parameters"=w304:T5)  [unwired: 11 in]
            n131 = for {
              tunnel: w304 -> [w310] mode=indexing
              tunnel: "Load output function" -> [w309]
              tunnel: [w308] -> w302 mode=indexing
              tunnel: [w307] -> w301 mode=indexing
              tunnel: [w306] -> w300 mode=indexing
              n132 = case shown="1006" w309 {
                tunnel: w310 -> [w314 w318]
                tunnel: [w313 w316] -> w308
                tunnel: [w312 w317] -> w307
                tunnel: [w311 w315] -> w306
                frame 1007, Default {
                  # "DC Current"
                  n133 = Unbundle By Name(w314) -> ("Current gain bandwidth"=w312:dbl, "Current compensation frequency"=w313:dbl, "Current pole-zero ratio"=w311:dbl)
                }
                frame 1006 {
                  # "DC Voltage"
                  n134 = Unbundle By Name(w318) -> ("Voltage gain bandwidth"=w317:dbl, "Voltage compensation frequency"=w316:dbl, "Voltage pole-zero ratio"=w315:dbl)
                }
              }
            }
            n135 = property on="Load voltage/current gain bandwidths" class="Arr (strict)"("Value"=w301) -> ()  [unwired: 2 in, 2 out]
            n136 = property on="Load voltage/current compensation frequencies" class="Arr (strict)"("Value"=w302) -> ()  [unwired: 2 in, 2 out]
            n137 = property on="Load voltage/current pole-zero ratios" class="Arr (strict)"("Value"=w300) -> ()  [unwired: 2 in, 2 out]
          }
          event Value Change {
            # "Legends view for voltage"
            n138 = event-data() -> ("NewVal"=w321:T1)  [unwired: 1 in]
            n139 = control-ref of="VoltageGraph"() -> (w322:refnum<vi>)
            n140 = case shown="True" w321 {
              tunnel: w322 -> [w326 w330]
              tunnel: w320 -> [w325 w328]
              tunnel: [w323 w327] -> w319
              frame False {
                # "Don't View Legend"
                n141 = property on="Property Node" class="WFGraph (strict)"(reference=w326, error in=w325, "Legend Visible"=FALSE ("Legend:Visible")) -> (error out=w323:errorcluster)  [unwired: 1 out]
              }
              frame True {
                w329 = TRUE ("Legend:Visible")
                # "View Legend"
                n142 = property on="Property Node" class="WFGraph (strict)"(reference=w330, error in=w328, "Legend Visible"=w329, "PlotVisCheckbox"=w329) -> (error out=w327:errorcluster)  [unwired: 1 out]
              }
            }
          }
          event Value Change {
            # "Legends view for current"
            n143 = event-data() -> ("NewVal"=w334:T1)  [unwired: 1 in]
            n144 = control-ref of="CurrentGraph"() -> (w331:refnum<vi>)
            n145 = case shown="False" w334 {
              tunnel: w331 -> [w338 w342]
              tunnel: w333 -> [w337 w340]
              tunnel: [w335 w339] -> w332
              frame False {
                # "Don't view legend"
                n146 = property on="Property Node" class="WFGraph (strict)"(reference=w338, error in=w337, "Legend Visible"=FALSE ("Legend:Visible")) -> (error out=w335:errorcluster)  [unwired: 1 out]
              }
              frame True {
                w341 = TRUE ("Legend:Visible")
                # "View legend"
                n147 = property on="Property Node" class="WFGraph (strict)"(reference=w342, error in=w340, "Legend Visible"=w341, "PlotVisCheckbox"=w341) -> (error out=w339:errorcluster)  [unwired: 1 out]
              }
            }
          }
          event Panel Close? {
            n148 = event-data() -> ()  [unwired: 1 in, 4 out]
            n149 = Enqueue Element(queue=w344, element="Exit", error in (no error)=w346) -> (error out=w345:errorcluster)  [unwired: 1 in, 2 out]
            n150 = event-data("Discard?"=TRUE) -> ()  [unwired: 1 in, 1 out]
          }
        }
      }
      frame "Initialize" {
        # "Initialization of controls or indicator if needed"
      }
      frame "Post UI Update" {
        w370 = 16 ("y")
        # "This case will be triggered, after framework updates the User interface with result values."
        n151 = local read "Ganged source voltages"() -> (w394:dbl[])
        n152 = local read "Ganged source currents"() -> (w395:dbl[])
        n153 = local read "Ganged load voltages"() -> (w359:dbl[])
        n154 = local read "Ganged load currents"() -> (w360:dbl[])
        n155 = local read "Source dt"() -> (w390:dbl[])
        n156 = local read "Load dt"() -> (w358:dbl[])
        n157 = Array Size(array=w390) -> (size(s)=w397:i32)
        n158 = Array Size(array=w394) -> (size(s)=w399:i32)
        n159 = Array Size(array=w395) -> (size(s)=w398:i32)
        n160 = Array Size(array=w359) -> (size(s)=w401:i32)
        n161 = Array Size(array=w360) -> (size(s)=w402:i32)
        n162 = Array Size(array=w358) -> (size(s)=w363:i32)
        n163 = local read "Source voltages"() -> (w393:dbl[])
        n164 = local read "Source currents"() -> (w384:dbl[])
        n165 = Index Array(array=w390) -> (element=w385:dbl)  [unwired: 1 in]
        n166 = Index Array(array=w358) -> (element=w357:dbl)  [unwired: 1 in]
        n167 = local read "Load voltages"() -> (w391:dbl[])
        n168 = local read "Load currents"() -> (w383:dbl[])
        n169 = To Double Precision Float(number=w397) -> (double precision float=w353:dbl)
        n170 = To Double Precision Float(number=w399) -> (double precision float=w356:dbl)
        n171 = To Double Precision Float(number=w398) -> (double precision float=w354:dbl)
        n172 = To Double Precision Float(number=w397) -> (double precision float=w355:dbl)
        n173 = To Double Precision Float(number=w401) -> (double precision float=w352:dbl)
        n174 = To Double Precision Float(number=w363) -> (double precision float=w351:dbl)
        n175 = To Double Precision Float(number=w402) -> (double precision float=w350:dbl)
        n176 = To Double Precision Float(number=w363) -> (double precision float=w349:dbl)
        n177 = Divide(x=w354, y=w353) -> (x/y=w396:dbl)
        n178 = Divide(x=w356, y=w355) -> (x/y=w400:dbl)
        n179 = Divide(x=w352, y=w351) -> (x/y=w362:dbl)
        n180 = Divide(x=w350, y=w349) -> (x/y=w361:dbl)
        n181 = for {
          N: w397 -> [_]
          tunnel: w400 -> [w461]
          shift-right: [w462] -> _
          shift-left: w394 -> [w463]
          tunnel: [w458] -> w381 mode=indexing
          tunnel: [w457] -> w380 mode=indexing
          shift-right: [w453] -> _
          shift-left: w395 -> [w454]
          tunnel: w396 -> [w452]
          tunnel: w390 -> [w451] mode=indexing
          n182 = To Long Integer(number=w461) -> (32bit integer=w450:i32)
          n183 = To Long Integer(number=w452) -> (32bit integer=w449:i32)
          n184 = Delete From Array(array=w463, length=w450, index=0) -> (deleted portion=w456:dbl[], array with subset deleted=w462:dbl[])
          n185 = Delete From Array(array=w454, length=w449, index=0) -> (deleted portion=w455:dbl[], array with subset deleted=w453:dbl[])
          n186 = Bundle By Name("dt"=w451, "Y"=w456) -> (w458:waveform(dbl))  [unwired: 1 in]
          n187 = Bundle By Name("dt"=w451, "Y"=w455) -> (w457:waveform(dbl))  [unwired: 1 in]
        }
        n188 = for {
          N: w363 -> [_]
          tunnel: w362 -> [w405]
          shift-right: [w416] -> _
          shift-left: w359 -> [w417]
          tunnel: [w413] -> w364 mode=indexing
          tunnel: [w412] -> w365 mode=indexing
          shift-right: [w408] -> _
          shift-left: w360 -> [w409]
          tunnel: w361 -> [w407]
          tunnel: w358 -> [w406] mode=indexing
          n189 = To Long Integer(number=w407) -> (32bit integer=w403:i32)
          n190 = To Long Integer(number=w405) -> (32bit integer=w404:i32)
          n191 = Delete From Array(array=w417, length=w404, index=0) -> (deleted portion=w411:dbl[], array with subset deleted=w416:dbl[])
          n192 = Delete From Array(array=w409, length=w403, index=0) -> (deleted portion=w410:dbl[], array with subset deleted=w408:dbl[])
          n193 = Bundle By Name("dt"=w406, "Y"=w411) -> (w413:waveform(dbl))  [unwired: 1 in]
          n194 = Bundle By Name("dt"=w406, "Y"=w410) -> (w412:waveform(dbl))  [unwired: 1 in]
        }
        n195 = Bundle By Name("dt"=w385, "Y"=w393) -> (w392:waveform(dbl))  [unwired: 1 in]
        n196 = Bundle By Name("dt"=w357, "Y"=w391) -> (w389:waveform(dbl))  [unwired: 1 in]
        n197 = Bundle By Name("dt"=w385, "Y"=w384) -> (w386:waveform(dbl))  [unwired: 1 in]
        n198 = Bundle By Name("dt"=w357, "Y"=w383) -> (w387:waveform(dbl))  [unwired: 1 in]
        n199 = Build Array("Source enable/disable", "Load enable/disable") -> (w375:bool[])
        n200 = Boolean Array To Number(Boolean array=w375) -> (number=w372:u32)
        n201 = case shown="1, Default" w372 {
          tunnel: w392 -> [w429 _]
          tunnel: w389 -> [_ w433]
          tunnel: [w427 w435] -> w388
          tunnel: w387 -> [_ w431]
          tunnel: w386 -> [w426 _]
          tunnel: [w424 w434] -> w382
          tunnel: w381 -> [w428 _]
          tunnel: w364 -> [_ w432]
          tunnel: w380 -> [w425 _]
          tunnel: w365 -> [_ w430]
          frame 1, Default {
            # "Source Enable"
            n202 = Build Array (concatenate)(w426, w425) -> (w424:waveform(dbl)[])
            n203 = Build Array (concatenate)(w429, w428) -> (w427:waveform(dbl)[])
          }
          frame 2 {
            # "Load Enable"
            n204 = Build Array (concatenate)(w431, w430) -> (w434:waveform(dbl)[])
            n205 = Build Array (concatenate)(w433, w432) -> (w435:waveform(dbl)[])
          }
        }
        "VoltageGraph" <- w388
        "CurrentGraph" <- w382
        n206 = case shown="2" w372 {
          tunnel: [w439 w441] -> w367
          frame 1, Default {
            # "Source Enable"
            n207 = property on="PPSResourceNames" class="Arr (strict)"() -> ("Value"=w436:refnum<k15>[])  [unwired: 2 in, 2 out]
            n208 = Insert Into Array(array=w436, index=0, new element="SystemSource" ("string")) -> (w439:refnum<k15>[])
          }
          frame 2 {
            # "Load Enable"
            n209 = property on="LoadResourceNames" class="Arr (strict)"() -> ("Value"=w440:refnum<k15>[])  [unwired: 2 in, 2 out]
            n210 = Insert Into Array(array=w440, index=0, new element="SystemLoad" ("string")) -> (w441:refnum<k15>[])
          }
        }
        n211 = Array Size(array=w367) -> (size(s)=w369:i32)
        n212 = Less?(x=w369, y=w370) -> (x < y?=w371:bool)
        n213 = Subtract(x=w370, y=w369) -> (x-y=w368:i32)
        n214 = case shown="True" w371 {
          tunnel: w368 -> [_ w422]
          tunnel: w367 -> [w418 w420]
          tunnel: [w418 w419] -> w366
          frame False {
            # "if more than 16 than it gives enough space"
          }
          frame True {
            # "for maintaining the UI legeneds symbols and names doesn't mix out"
            n215 = Initialize Array("" ("string"), w422) -> (w421:string[])
            n216 = Insert Into Array(array=w420, new element=w421) -> (w419:refnum<k15>[])  [unwired: 1 in]
          }
        }
        n217 = control-ref of="VoltageGraph"() -> (w379:refnum<vi>)
        n218 = control-ref of="CurrentGraph"() -> (w378:refnum<vi>)
        n219 = Build Array(w379, w378) -> (w377:refnum<vi>[])
        n220 = for {
          tunnel: w377 -> [w445] mode=indexing
          tunnel: w366 -> [w444]
          n221 = for {
            tunnel: w445 -> [w448]
            tunnel: w444 -> [w446] mode=indexing
            i -> [w447]
            n222 = property on="Property Node" class="WFGraph (strict)"(reference=w448, "Active Plot"=w447, "Plot.Plot Name"=w446) -> ()  [unwired: 1 in, 2 out]
          }
        }
      }
      frame "Exit" {
        # "This case is triggered to close the User Interface from framework"
        n223 = Flush Queue(queue=w468, error in (no error)=w470) -> (queue out=w467:refnum<queue>, error out=w466:errorcluster)  [unwired: 1 out]
        n224 = Release Queue(queue=w467, force destroy? (F)=TRUE, error in (no error)=w466) -> (error out=w465:errorcluster)  [unwired: 2 out]
      }
      frame "Handle Error" {
      }
    }
  }
